vi "Agilent 34970 Read Continuous.vi"(0 "VISA Resource Name":refnum<visa-resource-name>, 11 "error in (no error)":errorcluster) -> (4 "VISA resource name out":refnum<visa-resource-name>, 6 "Output Array":dbl[](array[numeric]) format="%.2f", 8 "read buffer":string, 15 "error out":errorcluster)   [LabVIEW 2020]
doc: "This VI lets you take simple temperature measurements. You can use various types of thermocouples, thermistors, or RTDs."
uses:
  Agilent 34970.lvlib
panel:
  in  "Byte Count (1024 bytes)":i32=1024
  out "return count":u32
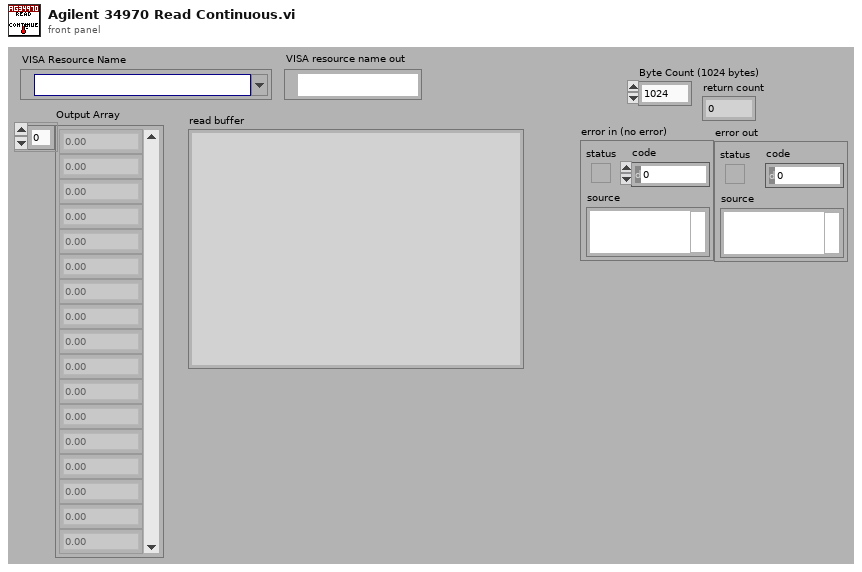
[diagram p1: front panel]
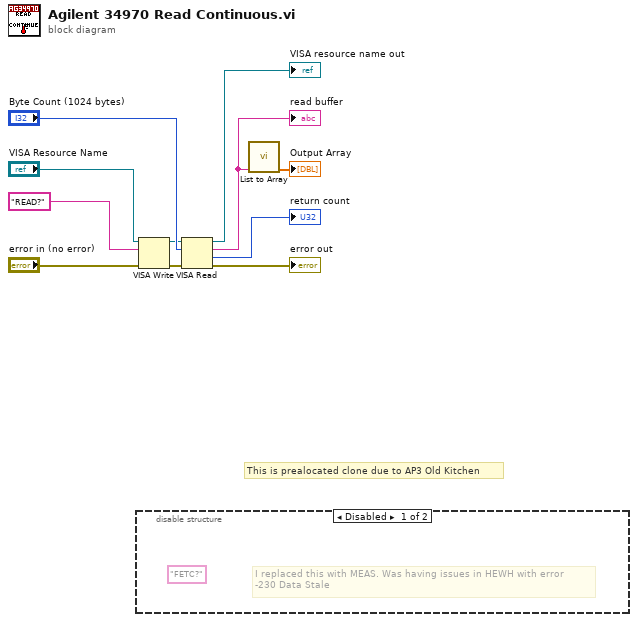
[diagram p0: block diagram]
diagram:
  # "This is prealocated clone due to AP3 Old Kitchen"
  n1 = disable-structure shown="Disabled" {
    frame Disabled {
      (unwired) "FETC?"
      # "I replaced this with MEAS. Was having issues in HEWH with error\n-230 Data Stale"
    }
    frame Enabled {
    }
  }
  n2 = VISA Write(VISA resource name="VISA Resource Name", write buffer="READ?", error in (no error)="error in (no error)") -> (VISA resource name out=w7:refnum<visa-resource-name>, error out=w8:errorcluster)  [unwired: 1 out]
  n3 = VISA Read(VISA resource name=w7, byte count="Byte Count (1024 bytes)", error in (no error)=w8) -> (VISA resource name out=→"VISA resource name out":refnum<visa-resource-name>, read buffer=w2:string, return count=→"return count":u32, error out=→"error out":errorcluster)
  "read buffer" <- w2
  n4 = call "List to Array.vi"("List (empty)"=w2) -> ("Output Number Array"=→"Output Array":dbl[])  [unwired: 9 in, 1 out]
